vi "central bead area.vi"(0 "Range (Threshold 1)":cluster{"Lower value":sgl, "Upper value":sgl}={"Lower value"=814.1775, "Upper value"=32767.0}, 1 "Keep/Remove Particles (Particle Filter 1)":bool=TRUE, 2 "Connectivity 4/8 (8) (Particle Filter 1)":bool=TRUE, 3 "Selection Values (Particle Filter 1)":T1(array[cluster]) {"Measurement Parameter" items=["Center of Mass X", "Center of Mass Y", "First Pixel X", "First Pixel Y", "Bounding Rect Left", "Bounding Rect Top", "Bounding Rect Right", "Bounding Rect Bottom", "Max Feret Diameter Start X", "Max Feret Diameter Start Y", "Max Feret Diameter End X", "Max Feret Diameter End Y", "Max Horiz. Segment Length Left", "Max Horiz. Segment Length Right", "Max Horiz. Segment Length Row", "-", "Bounding Rect Width", "Bounding Rect Height", "Bounding Rect Diagonal", "Perimeter", "Convex Hull Perimeter", "Holes' Perimeter", "Max Feret Diameter", "Equivalent Ellipse Major Axis", "Equivalent Ellipse Minor Axis", "Equivalent Ellipse Minor Axis (Feret)", "Equivalent Rect Long Side", "Equivalent Rect Short Side", "Equivalent Rect Diagonal", "Equivalent Rect Short Side (Feret)", "Average Horiz. Segment Length", "Average Vert. Segment Length", "Hydraulic Radius", "Waddel Disk Diameter", "-", "Area", "Holes' Area", "Particle & Holes' Area", "Convex Hull Area", "Image Area", "-", "Number of Holes", "Number of Horiz. Segments", "Number of Vert. Segments", "-", "Orientation", "Max Feret Diameter Orientation", "-", "% Area/Image Area", "% Area/(Particle & Holes' Area)", "Ratio of Equivalent Ellipse Axes", "Ratio of Equivalent Rect Sides", "-", "Elongation Factor", "Compactness Factor", "Heywood Circularity Factor", "Type Factor", "-", "Sum X", "Sum Y", "Sum XX", "Sum XY", "Sum YY", "Sum XXX", "Sum XXY", "Sum XYY", "Sum YYY", "-", "Moment of Inertia XX", "Moment of Inertia XY", "Moment of Inertia YY", "Moment of Inertia XXX", "Moment of Inertia XXY", "Moment of Inertia XYY", "Moment of Inertia YYY", "Norm. Moment of Inertia XX", "Norm. Moment of Inertia XY", "Norm. Moment of Inertia YY", "Norm. Moment of Inertia XXX", "Norm. Moment of Inertia XXY", "Norm. Moment of Inertia XYY", "Norm. Moment of Inertia YYY", "Hu Moment 1", "Hu Moment 2", "Hu Moment 3", "Hu Moment 4", "Hu Moment 5", "Hu Moment 6", "Hu Moment 7"]}, 4 "Number of Erosion (Advanced Morphology 1)":i32=2, 5 "Square/Hexa (Square) (Advanced Morphology 1)":bool, 6 "Connectivity 4/8 (8) (Advanced Morphology 1)":bool, 7 "error in":errorcluster, 8 "Low Pass/High Pass (Low) (Advanced Morphology 1)":bool, 9 "Connectivity 4/8 (8) (Particle Analysis 1)":bool=TRUE, 10 "Pixel Measurements (Particle Analysis 1)":i32[](array[ring])=[0, 1, 2, 3, 4, 5, 6, 7, 8, 9, 10, 11, 12, 13, 14, 16, 17, 18, 19, 20, 21, 22, 23, 24, 25, 26, 27, 28, 29, 30, 31, 32, 33, 35, 36, 37, 38, 39, 41, 42, 43, 45, 46, 48, 49, 50, 51, 53, 54, 55, 56, 58, 59, 60, 61, 62, 63, 64, 65, 66, 68, 69, 70, 71, 72, 73, 74, 75, 76, 77, 78, 79, 80, 81, 82, 83, 84, 85, 86, 87, 88] items=["Center of Mass X", "Center of Mass Y", "First Pixel X", "First Pixel Y", "Bounding Rect Left", "Bounding Rect Top", "Bounding Rect Right", "Bounding Rect Bottom", "Max Feret Diameter Start X", "Max Feret Diameter Start Y", "Max Feret Diameter End X", "Max Feret Diameter End Y", "Max Horiz. Segment Length Left", "Max Horiz. Segment Length Right", "Max Horiz. Segment Length Row", "-", "Bounding Rect Width", "Bounding Rect Height", "Bounding Rect Diagonal", "Perimeter", "Convex Hull Perimeter", "Holes' Perimeter", "Max Feret Diameter", "Equivalent Ellipse Major Axis", "Equivalent Ellipse Minor Axis", "Equivalent Ellipse Minor Axis (Feret)", "Equivalent Rect Long Side", "Equivalent Rect Short Side", "Equivalent Rect Diagonal", "Equivalent Rect Short Side (Feret)", "Average Horiz. Segment Length", "Average Vert. Segment Length", "Hydraulic Radius", "Waddel Disk Diameter", "-", "Area", "Holes' Area", "Particle & Holes' Area", "Convex Hull Area", "Image Area", "-", "Number of Holes", "Number of Horiz. Segments", "Number of Vert. Segments", "-", "Orientation", "Max Feret Diameter Orientation", "-", "% Area/Image Area", "% Area/(Particle & Holes' Area)", "Ratio of Equivalent Ellipse Axes", "Ratio of Equivalent Rect Sides", "-", "Elongation Factor", "Compactness Factor", "Heywood Circularity Factor", "Type Factor", "-", "Sum X", "Sum Y", "Sum XX", "Sum XY", "Sum YY", "Sum XXX", "Sum XXY", "Sum XYY", "Sum YYY", "-", "Moment of Inertia XX", "Moment of Inertia XY", "Moment of Inertia YY", "Moment of Inertia XXX", "Moment of Inertia XXY", "Moment of Inertia XYY", "Moment of Inertia YYY", "Norm. Moment of Inertia XX", "Norm. Moment of Inertia XY", "Norm. Moment of Inertia YY", "Norm. Moment of Inertia XXX", "Norm. Moment of Inertia XXY", "Norm. Moment of Inertia XYY", "Norm. Moment of Inertia YYY", "Hu Moment 1", "Hu Moment 2", "Hu Moment 3", "Hu Moment 4", "Hu Moment 5", "Hu Moment 6", "Hu Moment 7"], 11 "Real-World Measurements (Particle Analysis 1)":i32[](array[ring]) items=["Center of Mass X", "Center of Mass Y", "First Pixel X", "First Pixel Y", "Bounding Rect Left", "Bounding Rect Top", "Bounding Rect Right", "Bounding Rect Bottom", "Max Feret Diameter Start X", "Max Feret Diameter Start Y", "Max Feret Diameter End X", "Max Feret Diameter End Y", "Max Horiz. Segment Length Left", "Max Horiz. Segment Length Right", "Max Horiz. Segment Length Row", "-", "Bounding Rect Width", "Bounding Rect Height", "Bounding Rect Diagonal", "Perimeter", "Convex Hull Perimeter", "Holes' Perimeter", "Max Feret Diameter", "Equivalent Ellipse Major Axis", "Equivalent Ellipse Minor Axis", "Equivalent Ellipse Minor Axis (Feret)", "Equivalent Rect Long Side", "Equivalent Rect Short Side", "Equivalent Rect Diagonal", "Equivalent Rect Short Side (Feret)", "Average Horiz. Segment Length", "Average Vert. Segment Length", "Hydraulic Radius", "Waddel Disk Diameter", "-", "Area", "Holes' Area", "Particle & Holes' Area", "Convex Hull Area", "Image Area", "-", "Number of Holes", "Number of Horiz. Segments", "Number of Vert. Segments", "-", "Orientation", "Max Feret Diameter Orientation", "-", "% Area/Image Area", "% Area/(Particle & Holes' Area)", "Ratio of Equivalent Ellipse Axes", "Ratio of Equivalent Rect Sides", "-", "Elongation Factor", "Compactness Factor", "Heywood Circularity Factor", "Type Factor", "-", "Sum X", "Sum Y", "Sum XX", "Sum XY", "Sum YY", "Sum XXX", "Sum XXY", "Sum XYY", "Sum YYY", "-", "Moment of Inertia XX", "Moment of Inertia XY", "Moment of Inertia YY", "Moment of Inertia XXX", "Moment of Inertia XXY", "Moment of Inertia XYY", "Moment of Inertia YYY", "Norm. Moment of Inertia XX", "Norm. Moment of Inertia XY", "Norm. Moment of Inertia YY", "Norm. Moment of Inertia XXX", "Norm. Moment of Inertia XXY", "Norm. Moment of Inertia XYY", "Norm. Moment of Inertia YYY", "Hu Moment 1", "Hu Moment 2", "Hu Moment 3", "Hu Moment 4", "Hu Moment 5", "Hu Moment 6", "Hu Moment 7"], 12 "Min Radius (Circle Detection 1)":sgl=3.0, 13 "Max Radius (Circle Detection 1)":sgl=100.0) -> (20 "Number of Particles (Particle Analysis 1)":i32, 21 "Particle Measurements (Pixels) (Particle Analysis 1)":dbl[][](array[numeric]) format="%.2f", 22 "Particle Measurements (Real-World) (Particle Analysis 1)":dbl[][](array[numeric]) format="%.2f", 23 "Nb Circles (Circle Detection 1)":i32, 24 "Circles Data (Circle Detection 1)":T3(array[cluster]), 25 "Circles Data (calibrated) (Circle Detection 1)":T3(array[cluster]), 27 "error out":errorcluster)   [LabVIEW 2020]
uses:
  <vilib>/vision/NI_Vision_Development_Module.lvlib
panel:
  out "Image Out":T2(plugin-control)
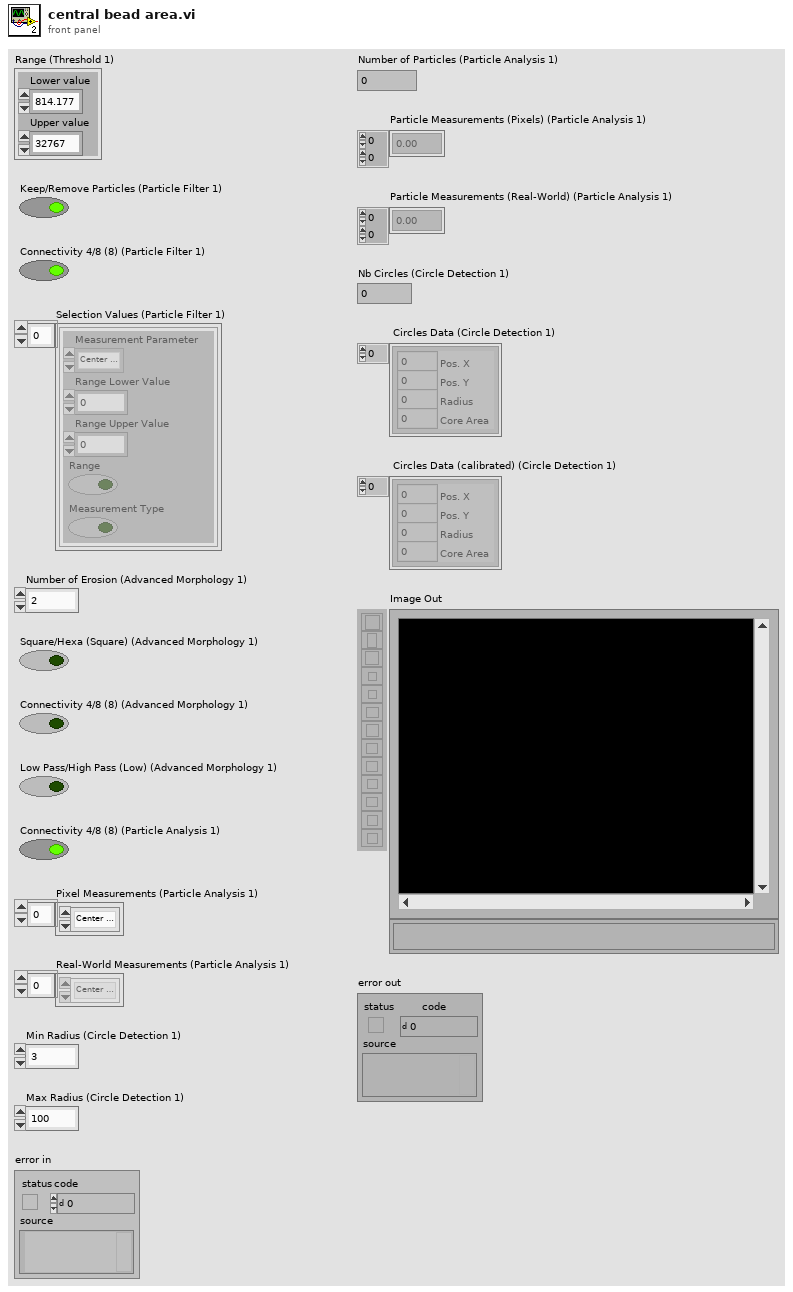
[diagram p1: front panel]
types:
  T1 = cluster{"Measurement Parameter":i32, "Range Lower Value":dbl, "Range Upper Value":dbl, "Range":bool, "Measurement Type":bool}[]
  T2 = typedef "IMAQ Image.ctl" = refnum<image>
  T3 = cluster{"Pos. X":i32, "Pos. Y":i32, "Radius":i32, "Core Area":i32}[]
  T4 = typedef "Image Type" = u32
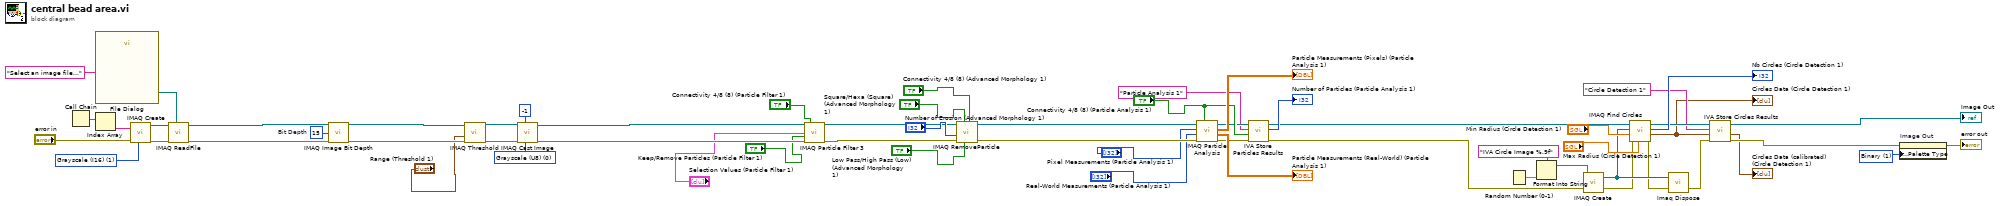
[diagram p0: block diagram]
diagram:
  w1 = u32 1 items=["Grayscale", "Binary", "Gradient", "Rainbow", "Temperature", "User Defined", "Binary 16 Bit", "Gradient 16 Bit", "Rainbow 16 Bit", "Temperature 16 Bit", "User Defined 16 Bit"] ("Palette Type")
  w41 = T4 0 items=["Grayscale (U8)", "Grayscale (I16)", "Grayscale (SGL)", "Complex (CSG)", "RGB (U32)", "HSL (U32)", "RGB (U64)", "Grayscale (U16)"] ("Image Type")
  w50 = u32 15  # Bit Depth
  w51 = T4 1 items=["Grayscale (U8)", "Grayscale (I16)", "Grayscale (SGL)", "Complex (CSG)", "RGB (U32)", "HSL (U32)", "RGB (U64)", "Grayscale (U16)"] ("Image Type")
  n1 = Call Chain() -> (call chain=w55:string[])
  n2 = Index Array(array=w55) -> (element=w54:string)  [unwired: 1 in]
  n3 = call "File Dialog"("prompt"="Select an image file...") -> ("selected path"=w52:path)  [unwired: 6 in, 8 out]
  n4 = call "IMAQ Create"("Image Name"=w54, "Image Type"=w51, "error in (no error)"="error in") -> ("New Image"=w58:T2, "error out"=w57:errorcluster)  [unwired: 1 in, 1 out]
  n5 = call "IMAQ ReadFile"("File Path"=w52, "error in (no error)"=w57, "Image"=w58) -> ("error out"=w59:errorcluster, "Image Out"=w49:T2)  [unwired: 2 in, 5 out]
  n6 = call "IMAQ Image Bit Depth"("Image"=w49, "Bit Depth (0)"=w50, "error in (no error)"=w59) -> ("Image Out"=w46:T2, "error out"=w48:errorcluster)  [unwired: 10 in, 1 out]
  n7 = call "IMAQ Threshold"("error in (no error)"=w48, "Range"="Range (Threshold 1)", "Image Src"=w46) -> ("error out"=w43:errorcluster, "Image Dst Out"=w44:T2)  [unwired: 3 in, 4 out]
  n8 = call "IMAQ Cast Image"("Image Type"=w41, "# Shifts"=-1, "error in (no error)"=w43, "Image Src"=w44) -> ("error out"=w45:errorcluster, "Image Dst Out"=w37:T2)  [unwired: 2 in, 4 out]
  n9 = call "IMAQ Particle Filter 3"("Image Src"=w37, "Connectivity 4/8 (8)"="Connectivity 4/8 (8) (Particle Filter 1)", "Selection Values"="Selection Values (Particle Filter 1)", "Keep/Remove Particles (F)"="Keep/Remove Particles (Particle Filter 1)", "error in (no error)"=w45) -> ("Image Dst Out"=w31:T2, "error out"=w38:errorcluster)  [unwired: 4 in, 5 out]
  n10 = call "IMAQ RemoveParticle"("Connectivity 4/8 (8)"="Connectivity 4/8 (8) (Advanced Morphology 1)", "Low Pass/High Pass (Low)"="Low Pass/High Pass (Low) (Advanced Morphology 1)", "Square/Hexa (Square)"="Square/Hexa (Square) (Advanced Morphology 1)", "error in (no error)"=w38, "Number of Erosion"="Number of Erosion (Advanced Morphology 1)", "Image Src"=w31) -> ("error out"=w30:errorcluster, "Image Dst Out"=w25:T2)  [unwired: 1 in, 3 out]
  n11 = call "IMAQ Particle Analysis"("Connectivity 4/8 (8)"="Connectivity 4/8 (8) (Particle Analysis 1)", "error in (no error)"=w30, "Real-World Measurements"="Real-World Measurements (Particle Analysis 1)", "Pixel Measurements"="Pixel Measurements (Particle Analysis 1)", "Image"=w25) -> ("error out"=w21:errorcluster, "Particle Measurements (Real-World)"=→"Particle Measurements (Real-World) (Particle Analysis 1)":dbl[][], "Particle Measurements (Pixels)"=→"Particle Measurements (Pixels) (Particle Analysis 1)":dbl[][], "Image Out (duplicate)"=w23:T2)  [unwired: 3 out]
  n12 = call <vilib>:"IVA Store Particles Results.vi"("error in (no error)"=w21, "Connectivity 4/8 (8)"="Connectivity 4/8 (8) (Particle Analysis 1)", "Step Name"="Particle Analysis 1", "Image in"=w23) -> ("error out"=w20:errorcluster, "Number of Particles"=→"Number of Particles (Particle Analysis 1)":i32, "Image dup"=w10:T2)  [unwired: 5 out]
  n13 = Random Number (0-1)() -> (number: 0 to 1=w4:dbl)
  n14 = Format Into String(format string="IVA Circle Image %.9f" ("Image Name"), w4) -> (resulting string=w6:string)  [unwired: 2 in, 1 out]
  n15 = call "IMAQ Create"("Image Name"=w6, "error in (no error)"=w20) -> ("New Image"=w15:T2, "error out"=w14:errorcluster)  [unwired: 2 in, 1 out]
  n16 = call "IMAQ Find Circles"("Max Radius"="Max Radius (Circle Detection 1)", "error in (no error)"=w14, "Min Radius"="Min Radius (Circle Detection 1)", "Image Dst"=w15, "Image Src"=w10) -> ("error out"=w13:errorcluster, "Circles Data"=w8:T3, "Nb Circles"=→"Nb Circles (Circle Detection 1)":i32)  [unwired: 4 out]
  "Circles Data (Circle Detection 1)" <- w8
  n17 = call "Imaq Dispose"("Image"=w15, "error in (no error)"=w13) -> ("error out"=w12:errorcluster)  [unwired: 1 in, 3 out]
  n18 = call <vilib>:"IVA Store Circles Results.vi"("error in (no error)"=w12, "Circles Data"=w8, "Step Name"="Circle Detection 1", "Image in"=w10) -> ("error out"=w11:errorcluster, "Circles Data (calibrated)"=→"Circles Data (calibrated) (Circle Detection 1)":T3, "Image dup"=→"Image Out":T2)  [unwired: 5 out]
  n19 = property on="Image Out" class="ImageControl"(error in=w11, "Palette:Palette Type"=w1) -> (error out=→"error out":errorcluster)  [unwired: 1 in, 1 out]
